vi "Worker.vi"(8 "Error In":errorcluster, 11 "Управление ПЛК вход":T1) -> (0 "Error Out":errorcluster, 3 "Управление ПЛК выход":T1)   [LabVIEW 2023, in "pump_Lib.lvlib"]
uses:
  pump_Lib.lvlib
  TypeDef/control_Type.ctl
  TypeDef/pump_Type.ctl
  TypeDef/pair_Type.ctl
  TypeDef/parametrs_Type.ctl
  <vilib>/Plasmionique/MB Master/MB_Master_TCP/MB_Master_TCP.lvclass
  C:/Program Files/National Instruments/LabVIEW 2023/vi.lib/Plasmionique/MB Master/MB_Master/MB_Master.lvclass
  <vilib>/Plasmionique/MB Master/MB Master.lvlib
panel:
  out "exit":bool
  out "result":bool
  out "Время цикла, мс":u32
  # "%"
  # "%"
  # "%"
  # "%"
  # "%"
  # "%"
  # "%"
  # "%"
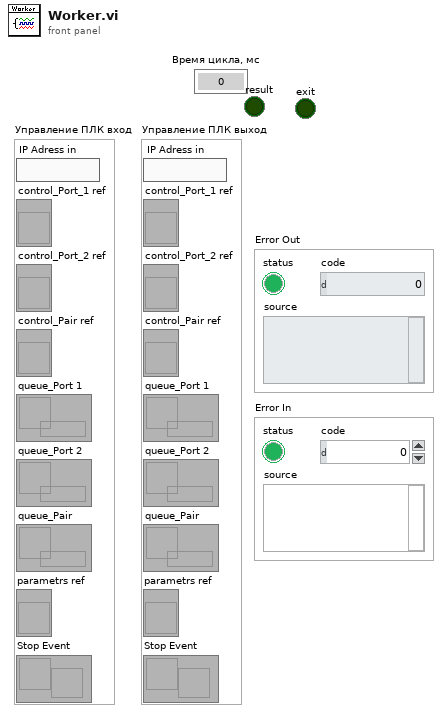
[diagram p1: front panel]
types:
  T1 = typedef "pump_Lib.lvlib/control_Type.ctl" = cluster{"IP Adress in":string, "control_Port_1 ref":refnum<vi>, "control_Port_2 ref":refnum<vi>, "control_Pair ref":refnum<vi>, "queue_Port 1":refnum<queue>, "queue_Port 2":refnum<queue>, "queue_Pair":refnum<queue>, "parametrs ref":refnum<vi>, "Stop Event":refnum<user-event>}
  T2 = typedef "pump_Lib.lvlib/pair_Type.ctl" = cluster{"Давление заданное":dbl, "Давление в системе":dbl, "Расход заданый":dbl, "Расход текущий":dbl, "Объём заданный":dbl, "Объём текущий":dbl, "Старт давление":bool, "Старт расход":bool, "Сброс объёма":bool, "plc_control":bool, "lag_control":bool, "mstop_control":bool, "Давление":cluster{"АЦП CH 0":dbl, "АЦП CH 1":dbl, "АЦП CH 2":dbl, "АЦП CH 3":dbl, "АЦП CH 4":dbl, "АЦП CH 5":dbl, "АЦП CH 6":dbl, "АЦП CH 7":dbl}, "Modbus":cluster{"Массив чтения":u16[], "Массив записи":u16[]}}
  T3 = typedef "pump_Lib.lvlib/pump_Type.ctl" = cluster{"Давление заданное":dbl, "Давление MAX заданное":dbl, "Давление в насосе":dbl, "Давление в системе":dbl, "Расход заданый":dbl, "Расход текущий":dbl, "Объём заданный":dbl, "Объём текущий":dbl, "Позиция насоса %":dbl, "Ток двигателя":dbl, "controlMsg":string, "Клапан k_sys":bool, "Клапан k_res":bool, "Клапан k_air":bool, "Вверх":bool, "Домой":bool, "Вниз":bool, "Старт расход":bool, "Старт давление":bool, "Сброс объёма":bool, "Сброс давления Рсис":bool, "Сброс давления Рнас":bool, "Bits":cluster{"plc_control":bool, "lag_control":bool, "mstop_control":bool, "st_home":bool, "error":bool, "mstart":bool, "pair":bool, "startQ":bool, "startP":bool, "volume_Stop":bool}}
  T4 = enum8{"Enabled", "Disabled", "Disabled and Grayed Out"}
  T5 = typedef "pump_Lib.lvlib/parametrs_Type.ctl" = cluster{"мл в час":bool, "Спарить насосы":bool, "DO-1":u16[]}
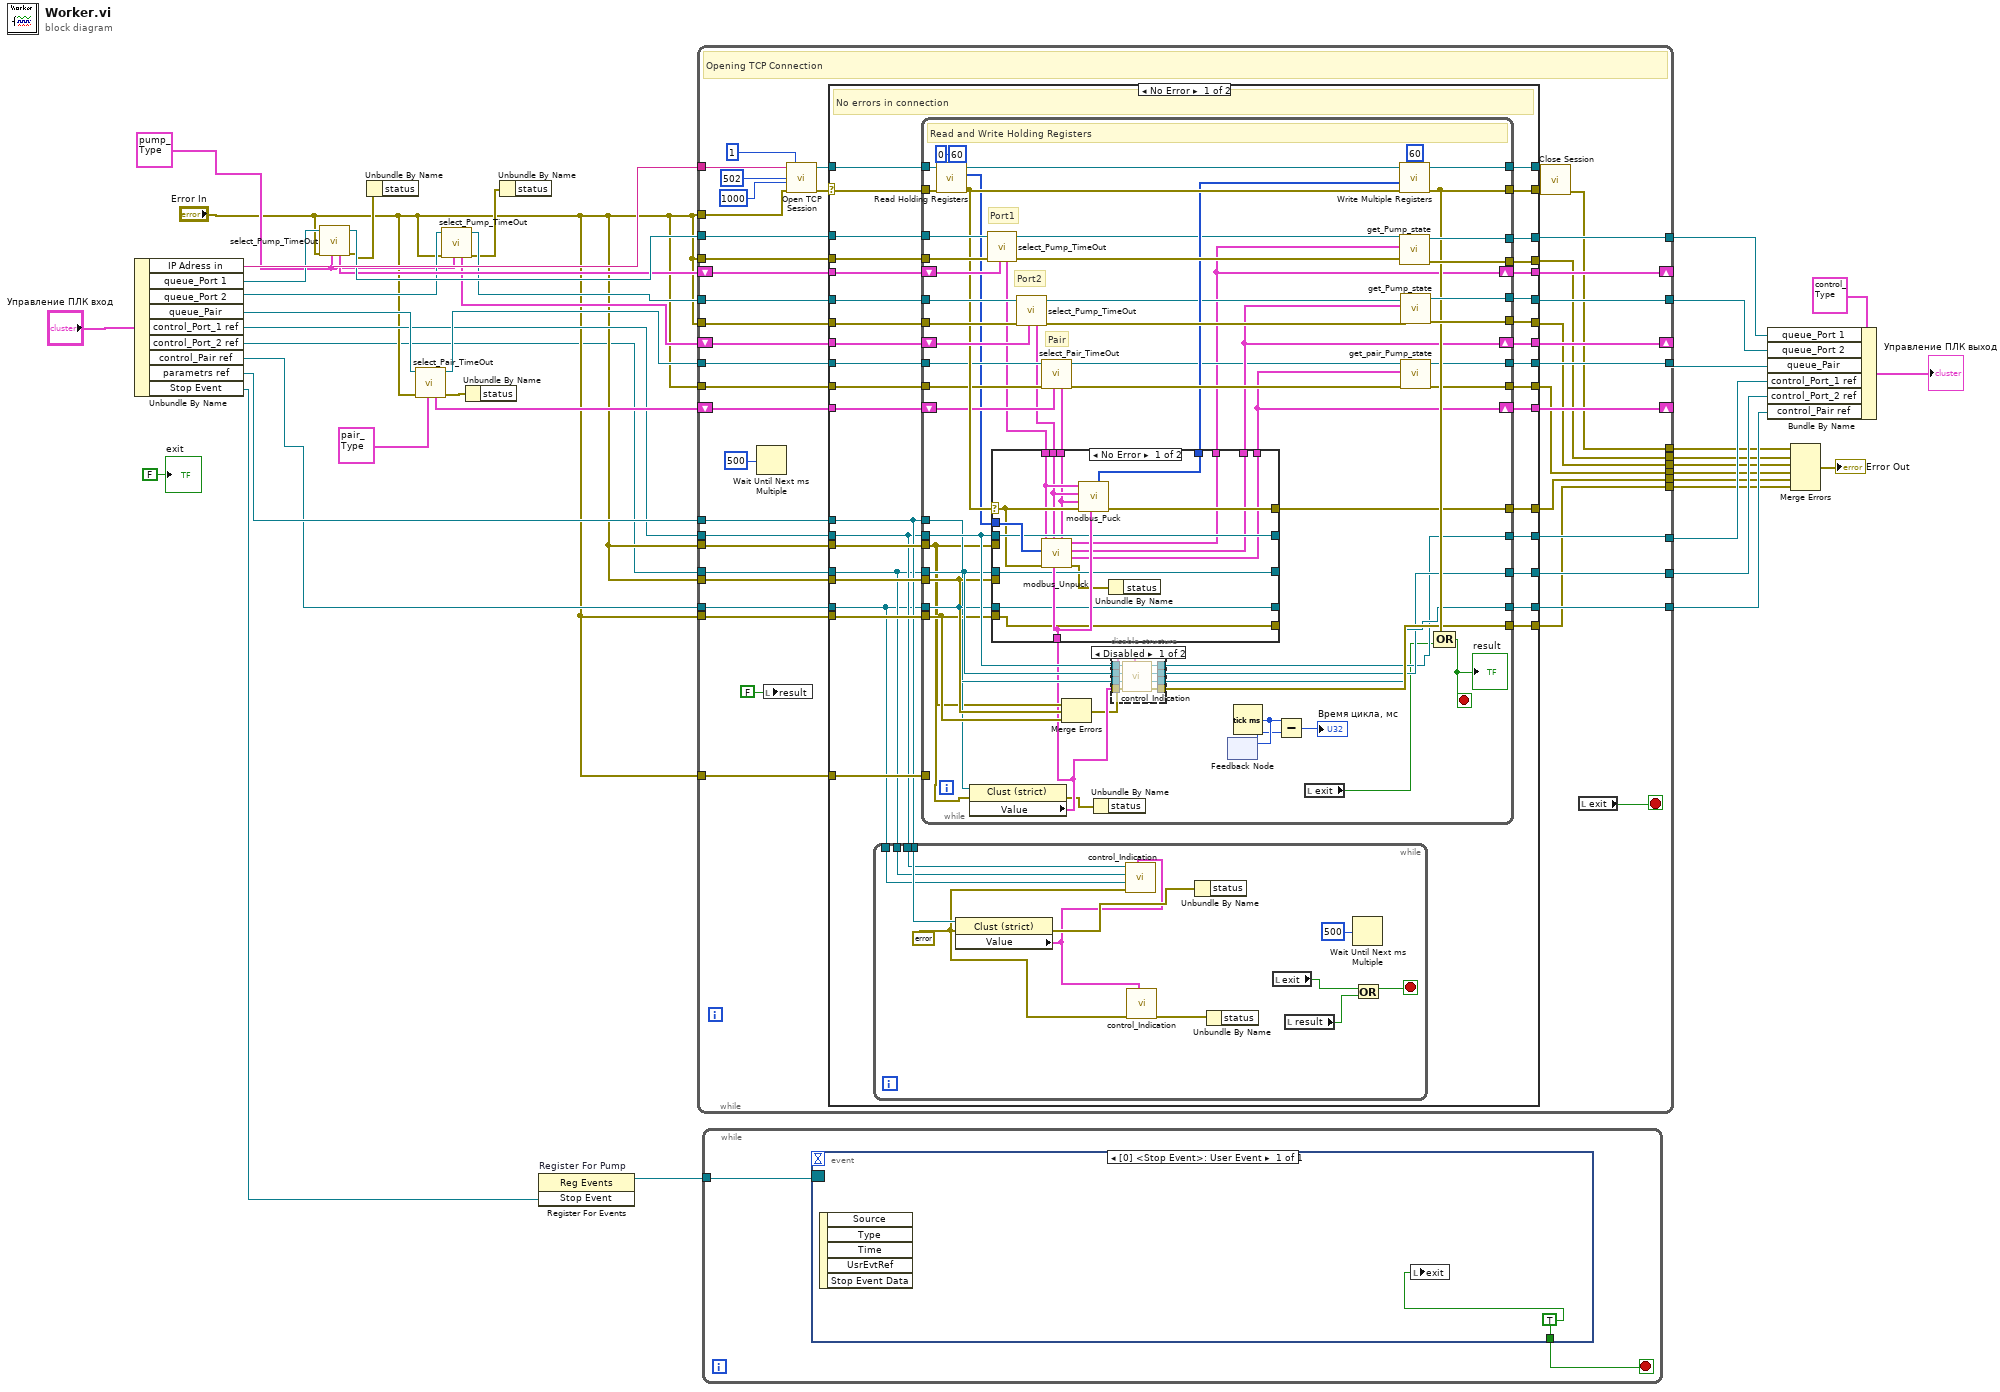
[diagram p0: block diagram]
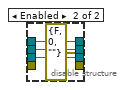
[diagram p2: hidden frame]
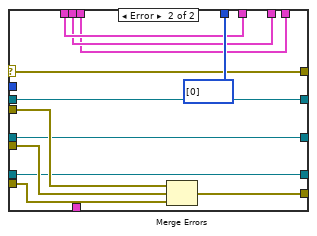
[diagram p3: hidden frame]
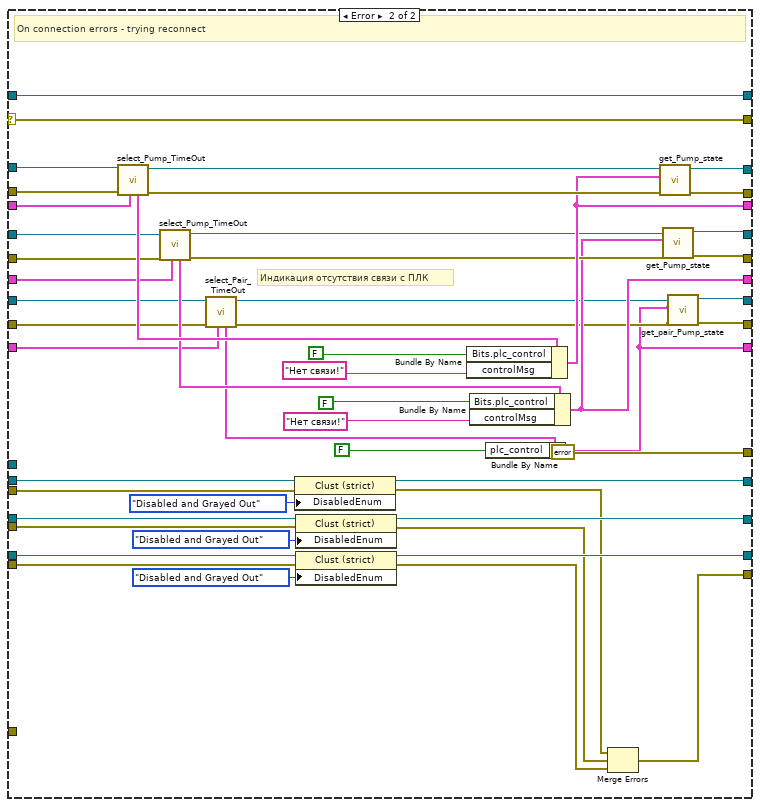
[diagram p4: hidden frame]
diagram:
  w16 = T3 {"Давление заданное"=0.3, "Давление MAX заданное"=100.0, "Давление в насосе"=0.0, "Давление в системе"=99.99, "Расход заданый"=0.0, "Расход текущий"=0.0, "Объём заданный"=0.0, "Объём текущий"=0.0, "Позиция насоса %"=0.0, "Ток двигателя"=0.0, "controlMsg"="", "Клапан k_sys"=FALSE, "Клапан k_res"=FALSE, "Клапан k_air"=FALSE, "Вверх"=FALSE, "Домой"=FALSE, "Вниз"=FALSE, "Старт расход"=FALSE, "Старт давление"=FALSE, "Сброс объёма"=FALSE, "Сброс давления Рсис"=FALSE, "Сброс давления Рнас"=FALSE, "Bits"={"plc_control"=FALSE, "lag_control"=FALSE, "mstop_control"=FALSE, "st_home"=FALSE, "error"=FALSE, "mstart"=FALSE, "pair"=FALSE, "startQ"=FALSE, "startP"=FALSE, "volume_Stop"=FALSE}} ("Насос")
  n1 = Unbundle By Name("Управление ПЛК вход") -> ("IP Adress in"=w39:string, "queue_Port 1"=w22:refnum<queue>, "queue_Port 2"=w19:refnum<queue>, "queue_Pair"=w13:refnum<queue>, "control_Port_1 ref"=w8:refnum<vi>, "control_Port_2 ref"=w4:refnum<vi>, "control_Pair ref"=w6:refnum<vi>, "parametrs ref"=w36:refnum<vi>, "Stop Event"=w1:refnum<user-event>)
  n2 = call "select_Pump_TimeOut.vi"("Насос in"=w16, "Error In"="Error In", "queue_Port in"=w22) -> ("Error Out"=w15:errorcluster, "queue_Port out"=w21:refnum<queue>, "Насос out"=w20:T3)  [unwired: 6 in]
  n3 = Unbundle By Name(w15) -> ()  [unwired: 1 out]
  n4 = call "select_Pair_TimeOut.vi"("Система in"=T2 {"Давление заданное"=0.3, "Давление в системе"=99.99, "Расход заданый"=0.0, "Расход текущий"=0.0, "Объём заданный"=0.0, "Объём текущий"=0.0, "Старт давление"=FALSE, "Старт расход"=FALSE, "Сброс объёма"=FALSE, "plc_control"=FALSE, "lag_control"=FALSE, "mstop_control"=FALSE, "Давление"={"АЦП CH 0"=0.0, "АЦП CH 1"=0.0, "АЦП CH 2"=0.0, "АЦП CH 3"=0.0, "АЦП CH 4"=0.0, "АЦП CH 5"=0.0, "АЦП CH 6"=0.0, "АЦП CH 7"=0.0}, "Modbus"={"Массив чтения"=[], "Массив записи"=[]}} ("Насосная система"), "Error In"="Error In", "queue_Pair in"=w13) -> ("Error Out"=w11:errorcluster, "queue_Pair out"=w12:refnum<queue>, "Система out"=w10:T2)  [unwired: 6 in]
  n5 = call "select_Pump_TimeOut.vi"("Насос in"=w16, "Error In"="Error In", "queue_Port in"=w19) -> ("Error Out"=w14:errorcluster, "queue_Port out"=w18:refnum<queue>, "Насос out"=w17:T3)  [unwired: 6 in]
  n6 = Unbundle By Name(w11) -> ()  [unwired: 1 out]
  n7 = Unbundle By Name(w14) -> ()  [unwired: 1 out]
  n8 = register-events "Register For Pump"(w1) -> (reference out=w2:refnum<event-registration>)  [unwired: 2 in, 1 out]
  n9 = while {
    tunnel: "Error In" -> [w82]
    tunnel: "Error In" -> [w79]
    tunnel: w21 -> [w78]
    tunnel: [w77] -> w35
    shift-right: [w57] -> _
    shift-left: w20 -> [w69]
    tunnel: w8 -> [w76]
    tunnel: "Error In" -> [w75]
    tunnel: [w66] -> w32
    tunnel: w18 -> [w74]
    tunnel: "Error In" -> [w73]
    shift-right: [w71] -> _
    shift-left: w17 -> [w72]
    tunnel: [w70] -> w34
    tunnel: w4 -> [w68]
    tunnel: "Error In" -> [w67]
    tunnel: [w65] -> w31
    tunnel: "Error In" -> [w63]
    tunnel: w39 -> [w62]
    tunnel: w6 -> [w56]
    tunnel: "Error In" -> [w55]
    tunnel: w12 -> [w54]
    tunnel: w36 -> [w49]
    shift-right: [w51] -> _
    shift-left: w10 -> [w52]
    tunnel: "Error In" -> [w53]
    tunnel: [w50] -> w33
    tunnel: [w48] -> w30
    tunnel: [w47] -> w29
    tunnel: [w46] -> w28
    tunnel: [w45] -> w27
    tunnel: [w44] -> w26
    tunnel: [w43] -> w24
    tunnel: [w42] -> w23
    stop <- w40 stop-if-true
    # "Opening TCP Connection"
    n10 = Wait Until Next ms Multiple(millisecond multiple=u32 500) -> ()  [unwired: 1 out]
    n11 = local write "result"(FALSE ("result")) -> ()
    n12 = call <vilib>:"Open TCP Session.vi"("Slave ID (255)"=u8 1, "error in (no error)"=w63, "Timeout (10000)"=1000, "Port (502)"=u16 502, "IP Address"=w62) -> ("error out"=w61:errorcluster, "MB_TCP session"=w60:refnum<class "MB_Master_TCP.lvclass">)  [unwired: 5 in]
    n13 = case shown="No Error" w61 {
      selector: w61 -> [w100 w277]
      tunnel: w82 -> [w118 w274]
      tunnel: w79 -> [w117 _]
      tunnel: w78 -> [w116 w275]
      tunnel: [w115 w242] -> w77
      tunnel: [w114 w241] -> w46
      tunnel: [w113 w240] -> w57
      tunnel: w69 -> [w103 w273]
      tunnel: w76 -> [w86 w266]
      tunnel: w75 -> [w112 w246]
      tunnel: [w107 w263] -> w66
      tunnel: w74 -> [w111 w271]
      tunnel: w73 -> [w110 w270]
      tunnel: w72 -> [w102 w269]
      tunnel: [w104 w236] -> w71
      tunnel: [w108 w238] -> w45
      tunnel: [w109 w239] -> w70
      tunnel: w68 -> [w85 w261]
      tunnel: w67 -> [w106 w262]
      tunnel: [w105 w260] -> w65
      tunnel: w60 -> [w101 w276]
      tunnel: [w99 w277] -> w59
      tunnel: [w98 w276] -> w58
      tunnel: w56 -> [w84 w259]
      tunnel: w55 -> [w97 w258]
      tunnel: [w96 w256] -> w48
      tunnel: [w95 w247] -> w42
      tunnel: w54 -> [w94 w255]
      tunnel: w53 -> [w93 w254]
      tunnel: w52 -> [w92 w253]
      tunnel: [w91 w231] -> w51
      tunnel: [w90 w234] -> w50
      tunnel: [w89 w233] -> w44
      tunnel: w49 -> [w87 _]
      tunnel: [w88 errorcluster {"status"=FALSE, "code"=0, "source"=""} ("error IO")] -> w43
      frame No Error {
        # "No errors in connection"
        n14 = while {
          tunnel: w87 -> [w130]
          tunnel: w86 -> [w129]
          tunnel: w85 -> [w128]
          tunnel: w84 -> [w127]
          stop <- w121 stop-if-true
          w123 = errorcluster {"status"=FALSE, "code"=0, "source"=""} ("error in (no error)")
          n15 = property class="Clust (strict)"(reference=w130, error in=w123) -> (error out=w126:errorcluster, "Value"=w124:T5)  [unwired: 1 out]
          n16 = call "control_Indication.vi"("Параметры"=w124, "Error In"=w123, "control_Pair ref in"=w127, "control_Port_2 ref in"=w128, "control_Port_1 ref in"=w129) -> ()  [unwired: 3 in, 4 out]
          n17 = call "control_Indication.vi"("Параметры"=w124, "Error In"=w123) -> ("Error Out"=w122:errorcluster)  [unwired: 6 in, 3 out]
          n18 = Unbundle By Name(w126) -> ()  [unwired: 1 out]
          n19 = Unbundle By Name(w122) -> ()  [unwired: 1 out]
          n20 = local read "exit"() -> (w119:bool)
          n21 = local read "result"() -> (w120:bool)
          n22 = Wait Until Next ms Multiple(millisecond multiple=u32 500) -> ()  [unwired: 1 out]
          n23 = Or(x=w119, y=w120) -> (x .or. y?=w121:bool)
        }
        n24 = while {
          tunnel: w118 -> [w176]
          tunnel: w117 -> [_]
          tunnel: w116 -> [w175]
          tunnel: [w187] -> w115
          tunnel: [w186] -> w114
          tunnel: w86 -> [w158]
          tunnel: w112 -> [w146]
          tunnel: w111 -> [w172]
          tunnel: w110 -> [w171]
          tunnel: [w185] -> w109
          tunnel: [w184] -> w108
          tunnel: [w136] -> w107
          tunnel: w85 -> [w157]
          tunnel: w106 -> [w156]
          tunnel: [w137] -> w105
          shift-right: [w140] -> w113
          shift-left: w103 -> [w173]
          shift-right: [w150] -> w104
          shift-left: w102 -> [w170]
          tunnel: w101 -> [w182]
          tunnel: w100 -> [w183]
          tunnel: [w168] -> w99
          tunnel: [w180] -> w98
          tunnel: w84 -> [w155]
          tunnel: w97 -> [w154]
          tunnel: [w138] -> w96
          tunnel: [w139] -> w95
          tunnel: w94 -> [w166]
          tunnel: w93 -> [w165]
          shift-right: [w149] -> w91
          shift-left: w92 -> [w164]
          tunnel: [w162] -> w90
          tunnel: [w161] -> w89
          tunnel: w87 -> [w147]
          tunnel: [w148] -> w88
          stop <- w188 stop-if-true
          # "Pair"
          # "Port2"
          # "Port1"
          # "Read and Write Holding Registers"
          n25 = call <vilib>:"Read Holding Registers.vi"("error in (no error)"=w183, "quantity"=u16 60, "starting address"=u16 0, "MB session in"=w182) -> ("error out"=w167:errorcluster, "Registers"=w159:u16[], "MB session out"=w181:refnum<class "MB_Master_TCP.lvclass">)  [unwired: 5 in]
          n26 = property class="Clust (strict)"(reference=w147, error in=w146) -> (error out=w144:errorcluster, "Value"=w145:T5)  [unwired: 1 out]
          n27 = call "select_Pump_TimeOut.vi"("Насос in"=w173, "Error In"=w176, "queue_Port in"=w175) -> ("Error Out"=w174:errorcluster, "queue_Port out"=w143:refnum<queue>, "Насос out"=w152:T3)  [unwired: 6 in]
          n28 = call "select_Pump_TimeOut.vi"("Насос in"=w170, "Error In"=w171, "queue_Port in"=w172) -> ("Error Out"=w169:errorcluster, "queue_Port out"=w142:refnum<queue>, "Насос out"=w153:T3)  [unwired: 6 in]
          n29 = call "select_Pair_TimeOut.vi"("Система in"=w164, "Error In"=w165, "queue_Pair in"=w166) -> ("Error Out"=w163:errorcluster, "queue_Pair out"=w141:refnum<queue>, "Система out"=w160:T2)  [unwired: 6 in]
          n30 = case shown="No Error" w167 {
            selector: w167 -> [w209 w218]
            tunnel: w160 -> [w206 w219]
            tunnel: w159 -> [w217 _]
            tunnel: w158 -> [w213 w226]
            tunnel: w146 -> [_ w229]
            tunnel: w157 -> [w212 w225]
            tunnel: w156 -> [_ w228]
            tunnel: w155 -> [w211 w223]
            tunnel: w154 -> [w210 w227]
            tunnel: w145 -> [w216 _]
            tunnel: w153 -> [w207 w220]
            tunnel: w152 -> [w208 w221]
            tunnel: [w210 w224] -> _
            tunnel: [w213 w226] -> _
            tunnel: [w212 w225] -> _
            tunnel: [w211 w223] -> _
            tunnel: [w215 u16[] [0] ("Modbus Write")] -> w151
            tunnel: [w205 w221] -> w140
            tunnel: [w204 w220] -> w150
            tunnel: [w203 w219] -> w149
            tunnel: [w214 w218] -> w148
            frame No Error {
              n31 = call "modbus_Unpuck.vi"("Pair in"=w206, "Параметры"=w216, "Port 2 in"=w207, "Error In"=w209, "Modbus Read"=w217, "Port 1 in"=w208) -> ("Error Out"=w202:errorcluster, "Pair out"=w203:T2, "Port 2 out"=w204:T3, "Port 1 out"=w205:T3)  [unwired: 2 in]
              n32 = call "modbus_Puck.vi"("Параметры"=w216, "Error In"=w209, "Pair in"=w206, "Port 2 in"=w207, "Port 1 in"=w208) -> ("Error Out"=w214:errorcluster, "Modbus Write"=w215:u16[])  [unwired: 2 in, 3 out]
              n33 = Unbundle By Name(w202) -> ()  [unwired: 1 out]
            }
            frame Error {
              n34 = Merge Errors(w229, w228, w227) -> (w224:errorcluster)
            }
          }
          n35 = Merge Errors(w146, w156, w154) -> (w135:errorcluster)
          n36 = Unbundle By Name(w144) -> ()  [unwired: 1 out]
          n37 = disable-structure shown="Disabled" {
            disable-tunnel: w158 -> [w197 w201]
            disable-tunnel: w157 -> [w196 w200]
            disable-tunnel: w155 -> [w195 w199]
            disable-tunnel: w145 -> [w194 _]
            disable-tunnel: [w193 errorcluster {"status"=FALSE, "code"=0, "source"=""} ("Error Out")] -> w139
            disable-tunnel: [w192 w199] -> w138
            disable-tunnel: [w191 w200] -> w137
            disable-tunnel: [w190 w201] -> w136
            disable-tunnel: w135 -> [w189 _]
            frame Disabled {
              n38 = call "control_Indication.vi"("Параметры"=w194, "Error In"=w189, "control_Pair ref in"=w195, "control_Port_2 ref in"=w196, "control_Port_1 ref in"=w197) -> ("Error Out"=w193:errorcluster, "control_Pair ref out"=w192:refnum<vi>, "control_Port_2 ref out"=w191:refnum<vi>, "control_Port_1 ref out"=w190:refnum<vi>)  [unwired: 3 in]
            }
            frame Enabled {
            }
          }
          n39 = feedback #1() -> (w133:u32)  [unwired: 1 in]
          n40 = Tick Count (ms)() -> (millisecond timer value=w134:u32)
          n41 = feedback-in #1(w134) -> ()
          n42 = Subtract(x=w134, y=w133) -> (x-y=→"Время цикла, мс":u32)
          n43 = local read "exit"() -> (w131:bool)
          n44 = call <vilib>:"Write Multiple Registers.vi"("error in (no error)"=w167, "values"=w151, "starting address"=u16 60, "MB session in"=w181) -> ("error out"=w168:errorcluster, "MB session out"=w180:refnum<class "MB_Master_TCP.lvclass">)  [unwired: 6 in]
          n45 = call "get_Pump_state.vi"("Error In"=w174, "Насос in"=w140, "queue_Port in"=w143) -> ("Error Out"=w186:errorcluster, "queue_Port out"=w187:refnum<queue>)  [unwired: 7 in]
          n46 = call "get_Pump_state.vi"("Error In"=w169, "Насос in"=w150, "queue_Port in"=w142) -> ("Error Out"=w184:errorcluster, "queue_Port out"=w185:refnum<queue>)  [unwired: 7 in]
          n47 = call "get_pair_Pump_state.vi"("Error In"=w163, "Система in"=w149, "queue_Pair in"=w141) -> ("Error Out"=w161:errorcluster, "queue_Pair out"=w162:refnum<queue>)  [unwired: 7 in]
          n48 = Compound Arithmetic op=OR(w168, w131) -> (w188:bool)
          "result" <- w188
        }
      }
      frame Error {
        # "Индикация отсутствия связи с ПЛК"
        # "On connection errors - trying reconnect"
        n49 = call "select_Pump_TimeOut.vi"("Насос in"=w273, "Error In"=w274, "queue_Port in"=w275) -> ("Error Out"=w243:errorcluster, "queue_Port out"=w244:refnum<queue>, "Насос out"=w272:T3)  [unwired: 6 in]
        n50 = call "select_Pump_TimeOut.vi"("Насос in"=w269, "Error In"=w270, "queue_Port in"=w271) -> ("Error Out"=w237:errorcluster, "queue_Port out"=w235:refnum<queue>, "Насос out"=w268:T3)  [unwired: 6 in]
        n51 = call "select_Pair_TimeOut.vi"("Система in"=w253, "Error In"=w254, "queue_Pair in"=w255) -> ("Error Out"=w232:errorcluster, "queue_Pair out"=w230:refnum<queue>, "Система out"=w252:T2)  [unwired: 6 in]
        n52 = property class="Clust (strict)"(reference=w266, error in=w246, "DisabledEnum"=T4."Disabled and Grayed Out" ("Disabled")) -> (reference out=w263:refnum<vi>, error out=w250:errorcluster)
        n53 = property class="Clust (strict)"(reference=w261, error in=w262, "DisabledEnum"=T4."Disabled and Grayed Out" ("Disabled")) -> (reference out=w260:refnum<vi>, error out=w249:errorcluster)
        n54 = property class="Clust (strict)"(reference=w259, error in=w258, "DisabledEnum"=T4."Disabled and Grayed Out" ("Disabled")) -> (reference out=w256:refnum<vi>, error out=w248:errorcluster)
        n55 = Bundle By Name(cluster=w272, "Bits.plc_control"=FALSE ("PLC"), "controlMsg"="Нет связи!") -> (w240:T3)
        n56 = Bundle By Name(cluster=w268, "Bits.plc_control"=FALSE ("PLC"), "controlMsg"="Нет связи!") -> (w236:T3)
        n57 = Bundle By Name(cluster=w252, "plc_control"=FALSE) -> (w231:T2)
        n58 = Merge Errors(w250, w249, w248) -> (w247:errorcluster)
        n59 = call "get_Pump_state.vi"("Error In"=w243, "Насос in"=w240, "queue_Port in"=w244) -> ("Error Out"=w241:errorcluster, "queue_Port out"=w242:refnum<queue>)  [unwired: 7 in]
        n60 = call "get_Pump_state.vi"("Error In"=w237, "Насос in"=w236, "queue_Port in"=w235) -> ("Error Out"=w238:errorcluster, "queue_Port out"=w239:refnum<queue>)  [unwired: 7 in]
        n61 = call "get_pair_Pump_state.vi"("Error In"=w232, "Система in"=w231, "queue_Pair in"=w230) -> ("Error Out"=w233:errorcluster, "queue_Pair out"=w234:refnum<queue>)  [unwired: 7 in]
      }
    }
    n62 = call-dynamic "Close Session.vi"("error in (no error)"=w59, "MB TCP session"=w58) -> ("error out"=w47:errorcluster)  [unwired: 9 in]
    n63 = local read "exit"() -> (w40:bool)
  }
  n64 = while {
    tunnel: w2 -> [w281]
    stop <- w282 stop-if-true
    n65 = event shown="[0] <Stop Event>: User Event" {
      selector: w281 -> [_]
      dyn-events: _ -> [_]
      timeout: _ -> [_]
      tunnel: [w283] -> w282
      event User Event {
        w283 = TRUE
        n66 = event-data() -> ()  [unwired: 1 in, 5 out]
        n67 = local write "exit"(w283) -> ()
      }
    }
  }
  n68 = Bundle By Name(cluster=T1 {"IP Adress in"="", "control_Port_1 ref"=refnum, "control_Port_2 ref"=refnum, "control_Pair ref"=refnum, "queue_Port 1"=refnum, "queue_Port 2"=refnum, "queue_Pair"=refnum, "parametrs ref"=refnum, "Stop Event"=refnum} ("Управление ПЛК выход 2"), "queue_Port 1"=w35, "queue_Port 2"=w34, "queue_Pair"=w33, "control_Port_1 ref"=w32, "control_Port_2 ref"=w31, "control_Pair ref"=w30) -> (→"Управление ПЛК выход":T1)
  n69 = Merge Errors(w29, w28, w27, w26, w24, w23) -> (→"Error Out":errorcluster)
  "exit" <- FALSE ("exit")
